vi "Periodic Tasks.vi"(8 "error in":errorcluster) -> ()   [LabVIEW 2014]
doc: "This VI runs in parallel to other tasks. It can contain as many user-defined periodic loops as you need. These can carry out PID or other sorts of timed response."
uses:
  Nav6Library/Nav6.lvlib
  <vilib>/addons/control/pid/NI_PID_pid.lvlib
  <vilib>/addons/control/pid/pid.llb/PID Advanced (DBL).vi
panel:
  in  "PID gains":T1={"proportional gain (Kc)"=1.0, "integral time (Ti, min)"=0.01, "derivative time (Td, min)"=0.0} {"derivative time (Td, min)" format="%.3f"; "integral time (Ti, min)" format="%.3f"; "proportional gain (Kc)" format="%.3f"}
  in  "output range":cluster{"output high":dbl, "output low":dbl}={"output high"=100.0, "output low"=-100.0} {"output low" format="%.2f"; "output high" format="%.2f"}
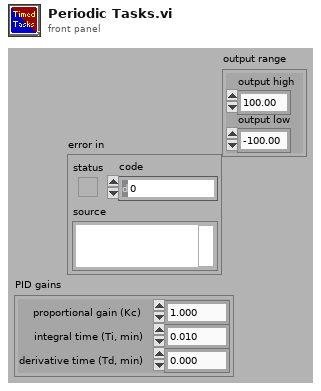
[diagram p1: front panel]
types:
  T1 = cluster{"proportional gain (Kc)":dbl, "integral time (Ti, min)":dbl, "derivative time (Td, min)":dbl}
  T2 = cluster{"notifier out":refnum<notifier>, "EoT?":bool, "Setpoint":dbl, "Manual Control":bool}
  T3 = typedef "Nav6.lvlib/Nav6DevRef.ctl" = cluster{"SerialPortRef":T4, "UpdateRate":u8, "Error":errorcluster, "Nav6Mode":T5}
  T4 = typedef "WPI_SerialPortRef.ctl" = cluster{"DevStatus":errorcluster, "Serial Port Name":refnum<visa-resource-name>}
  T5 = typedef "Nav6.lvlib/Nav6Mode.ctl" = enum16{"YPR", "Gyro", "Quaternion"}
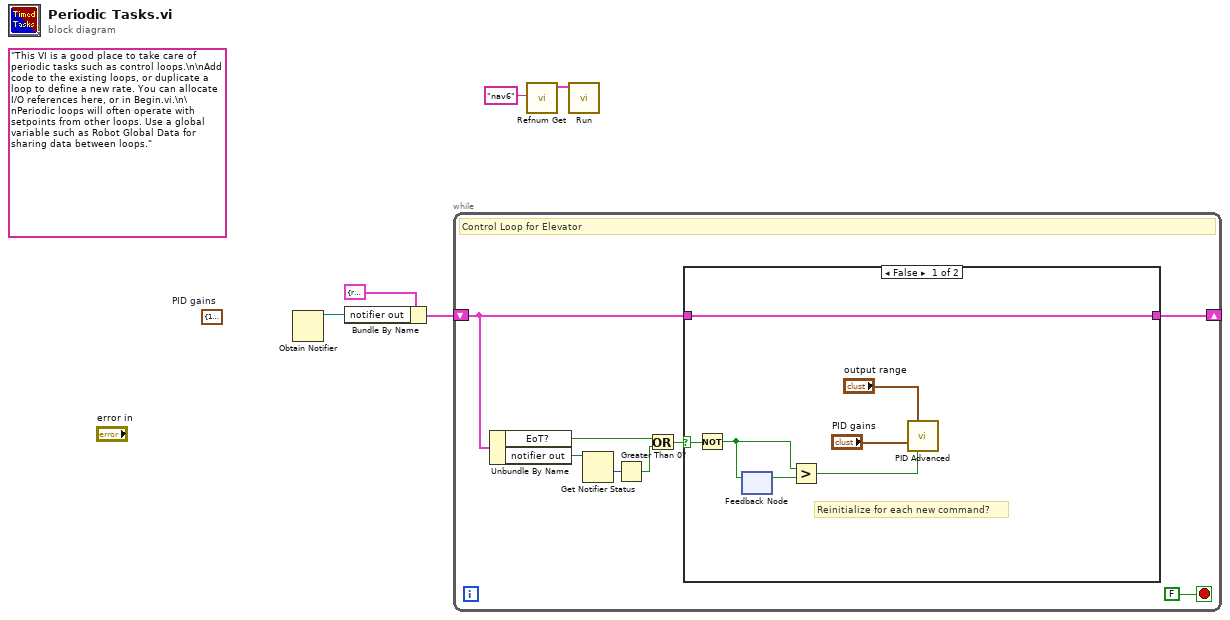
[diagram p0: block diagram]
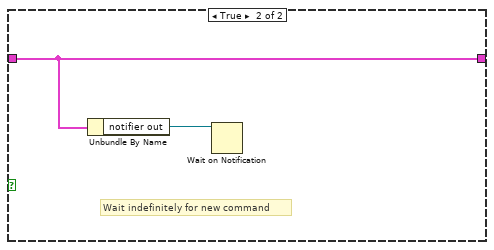
[diagram p2: hidden frame]
diagram:
  (unwired) T1 {"proportional gain (Kc)"=1.0, "integral time (Ti, min)"=0.01, "derivative time (Td, min)"=0.0}  # PID gains
  (unwired) "This VI is a good place to take care of periodic tasks such as control loops.\n\nAdd code to the existing loops, or duplicate a loop to define a new rate. You can allocate I/O references here, or in Begin.vi.\n\nPeriodic loops will often operate with setpoints from other loops. Use a global variable such as Robot Global Data for sharing data between loops."
  n1 = Obtain Notifier() -> (notifier out=w1:refnum<notifier>)  [unwired: 4 in, 2 out]
  n2 = Bundle By Name(cluster=T2 {"notifier out"=refnum, "EoT?"=TRUE, "Setpoint"=0.0, "Manual Control"=TRUE}, "notifier out"=w1) -> (w2:T2)
  n3 = while {
    shift-right: [w13] -> _
    shift-left: w2 -> [w12]
    stop <- FALSE stop-if-true
    # "Control Loop for Elevator"
    n4 = Unbundle By Name(w12) -> ("EoT?"=w8:bool, "notifier out"=w11:refnum<notifier>)
    n5 = Get Notifier Status(notifier=w11) -> (# waiting=w10:i32)  [unwired: 1 in, 4 out]
    n6 = Greater Than 0?(x=w10) -> (x > 0?=w9:bool)
    n7 = Or(x=w8, y=w9) -> (x .or. y?=w7:bool)
    n8 = case shown="False" w7 {
      selector: w7 -> [w17 _]
      tunnel: w12 -> [w20 w21]
      tunnel: [w20 w21] -> w13
      frame False {
        # "Reinitialize for each new command?"
        n9 = Not(x=w17) -> (.not. x?=w16:bool)
        n10 = feedback-in #1(w16) -> ()
        n11 = feedback #1() -> (w15:bool)  [unwired: 1 in]
        n12 = Greater?(x=w16, y=w15) -> (0:w14:bool)
        n13 = call-poly <vilib>:"PID Advanced.vi"("output range"="output range", "PID gains"="PID gains", "reinitialize? (F)"=w14) -> ()  [unwired: 11 in, 2 out]
      }
      frame True {
        # "Wait indefinitely for new command"
        n14 = Unbundle By Name(w21) -> ("notifier out"=w22:refnum<notifier>)
        n15 = Wait on Notification(notifier=w22) -> ()  [unwired: 3 in, 4 out]
      }
    }
  }
  n16 = call "Refnum Get.vi"("refnum name"="nav6") -> ("Nav6DevRef"=w4:T3)  [unwired: 9 in, 1 out]
  n17 = call "Run.vi"("Nav6DevRef"=w4) -> ()  [unwired: 11 in]
